vi "Handle Token Response.vi"(8 "error in (no error)":errorcluster, 10 "Response Body":string, 11 "Async Authorization in":refnum<class "Async Authorization.lvclass">) -> (0 "error out":errorcluster, 3 "Asyn Authorization out":refnum<class "Async Authorization.lvclass">)   [LabVIEW 2020, in "OAuth2.lvlib" / "Async Authorization.lvclass"]
uses:
  Async Authorization.lvclass
  Async Authorization.lvclass/Async Authorization.ctl
  Authorization/Authorization.lvclass
  <vilib>/JDP Science/JSONtext/JSONtext.lvlib
  3b40fd08-d5a5-4162-adab-a042d9031a6d.vi
  OAuth2.lvlib
  OAuth2 Error.ctl
  91bfb698-6b5f-49b7-b38b-bb1205cacc3f.vi
  6fcb67e5-1c0f-4de0-b6c6-12c162a38339.vi
  0bea330e-9405-428d-bd48-17c5eec9d49e.vi
  95191049-1c71-4619-a603-7357aa15aef9.vi
  7df24fda-659b-4cad-8c70-57ba007ebb44.vi
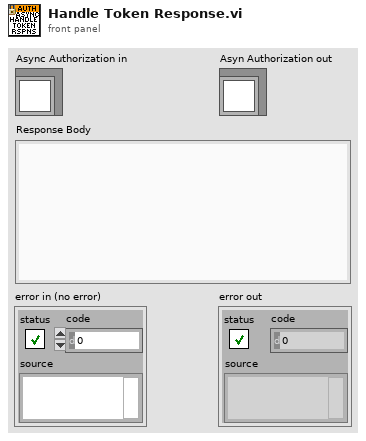
[diagram p1: front panel]
types:
  T1 = typedef "OAuth2.lvlib/OAuth2 Error.ctl" = enum16{"no_error", "admin_policy_enforced", "disallowed_useragent", "org_internal", "invalid_grant", "redirect_uri_mismatch", "invalid_request", "access_denied"}
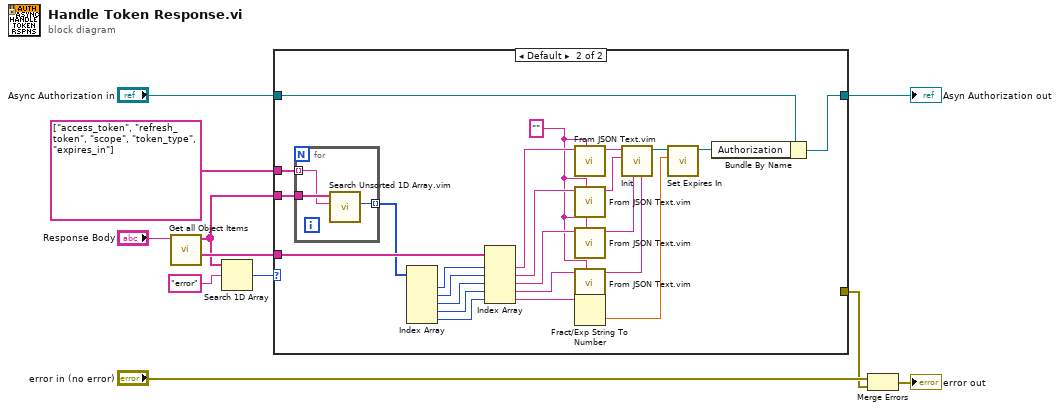
[diagram p0: block diagram]
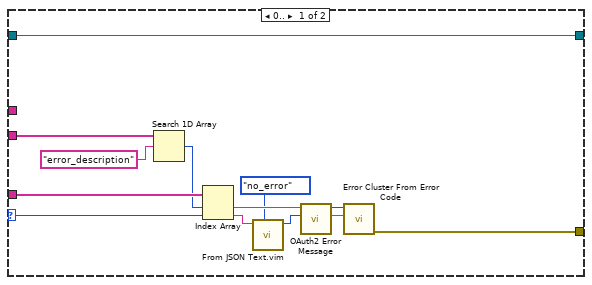
[diagram p2: hidden frame]
diagram:
  n1 = call <vilib>:"Get all Object Items.vi"("JSON"="Response Body") -> ("<JSON>"=w8:string[], "Item Names"=w5:string[])  [unwired: 7 in, 2 out]
  n2 = Search 1D Array(1D array=w5, element="error" ("String")) -> (index of element=w3:i32)  [unwired: 1 in]
  n3 = case shown="Default" w3 {
    selector: w3 -> [w20 _]
    tunnel: "Async Authorization in" -> [w24 w44]
    tunnel: [w24 w43] -> w9
    tunnel: w8 -> [w21 w42]
    tunnel: string[] ["access_token", "refresh_token", "scope", "token_type", "expires_in"] ("Search Keys") -> [_ w41]
    tunnel: w5 -> [w23 w26]
    tunnel: [w15 _] -> w1
    frame 0.. {
      n4 = Search 1D Array(1D array=w23, element="error_description" ("String")) -> (index of element=w19:i32)  [unwired: 1 in]
      n5 = Index Array(array=w21, index #1=w19, index #2=w20) -> (element #1=w18:string, element #2=w14:string)
      n6 = call "From JSON Text.vim"("Data Type and Default Value"=OAuth2_Error."no_error" ("OAuth2 Error"), "JSON"=w14) -> ("Data out"=w12:T1)  [unwired: 8 in, 1 out]
      n7 = call "OAuth2 Error Message.vi"("OAuth2 Error"=w12, "error_description"=w18) -> ("Error Message"=w16:string, "Error Code"=w17:i32)  [unwired: 8 in]
      n8 = call <vilib>:"Error Cluster From Error Code.vi"("error message (\"\")"=w16, "error code (0)"=w17) -> ("error out"=w15:errorcluster)  [unwired: 7 in]
    }
    frame Default {
      w25 = ""
      n9 = for {
        tunnel: w26 -> [w51]
        tunnel: w41 -> [w50] mode=indexing
        tunnel: [w49] -> w40 mode=indexing
        n10 = call "Search Unsorted 1D Array.vim"("element"=w50, "unsorted 1D array"=w51) -> ("index of element"=w49:i32)  [unwired: 9 in]
      }
      n11 = Index Array(array=w40) -> (element #1=w39:i32, element #2=w38:i32, element #3=w37:i32, element #4=w36:i32, element #5=w35:i32)  [unwired: 5 in]
      n12 = Index Array(array=w42, index #1=w39, index #2=w38, index #3=w37, index #4=w36, index #5=w35) -> (element #1=w34:string, element #2=w31:string, element #3=w32:string, element #4=w33:string, element #5=w48:string)
      n13 = call "From JSON Text.vim"("Data Type and Default Value"=w25, "JSON"=w34) -> ("Data out"=w30:string)  [unwired: 8 in, 1 out]
      n14 = call "From JSON Text.vim"("Data Type and Default Value"=w25, "JSON"=w31) -> ("Data out"=w29:string)  [unwired: 8 in, 1 out]
      n15 = call "From JSON Text.vim"("Data Type and Default Value"=w25, "JSON"=w32) -> ("Data out"=w28:string)  [unwired: 8 in, 1 out]
      n16 = call "From JSON Text.vim"("Data Type and Default Value"=w25, "JSON"=w33) -> ("Data out"=w27:string)  [unwired: 8 in, 1 out]
      n17 = Fract/Exp String To Number(string=w48) -> (number=w46:dbl)  [unwired: 3 in, 1 out]
      n18 = call "Init.vi"("Token Type"=w27, "Scope"=w28, "Refresh Token"=w29, "Access Token"=w30) -> ("Authorization"=w47:refnum<class "Authorization.lvclass">)  [unwired: 7 in]
      n19 = call "Set Expires In.vi"("Expires In"=w46, "Authorization in"=w47) -> ("Authorization out"=w45:refnum<class "Authorization.lvclass">)  [unwired: 9 in]
      n20 = Bundle By Name(cluster=w44, "Authorization"=w45) -> (w43:refnum<class "Async Authorization.lvclass">)
    }
  }
  "Asyn Authorization out" <- w9
  n21 = Merge Errors("error in (no error)", w1) -> (→"error out":errorcluster)
